vi "DOE Extract TCs.vi"(6 "Data Logger Type":T1=enum."Agilent", 8 "Error In":errorcluster, 9 "Agilent Array":dbl[](array[numeric]), 10 "TC Coefficients":T2, 11 "Kitchen Cluster in":T3) -> (0 "Error Out":errorcluster, 2 "TC Coefficients Out":T2, 3 "Kitchen Cluster out":T3, 4 "appended array":i32[](array[numeric]))   [LabVIEW 2018]
uses:
  Type Definitions/DOE Kitchen Control.ctl
  Utility/Type Definitions/UTILITY TC Coefficients.ctl
  Type Definitions/DOE Data Logger Type.ctl
  Utility/Type Definitions/UTILITY TC Coefficients Selector.ctl
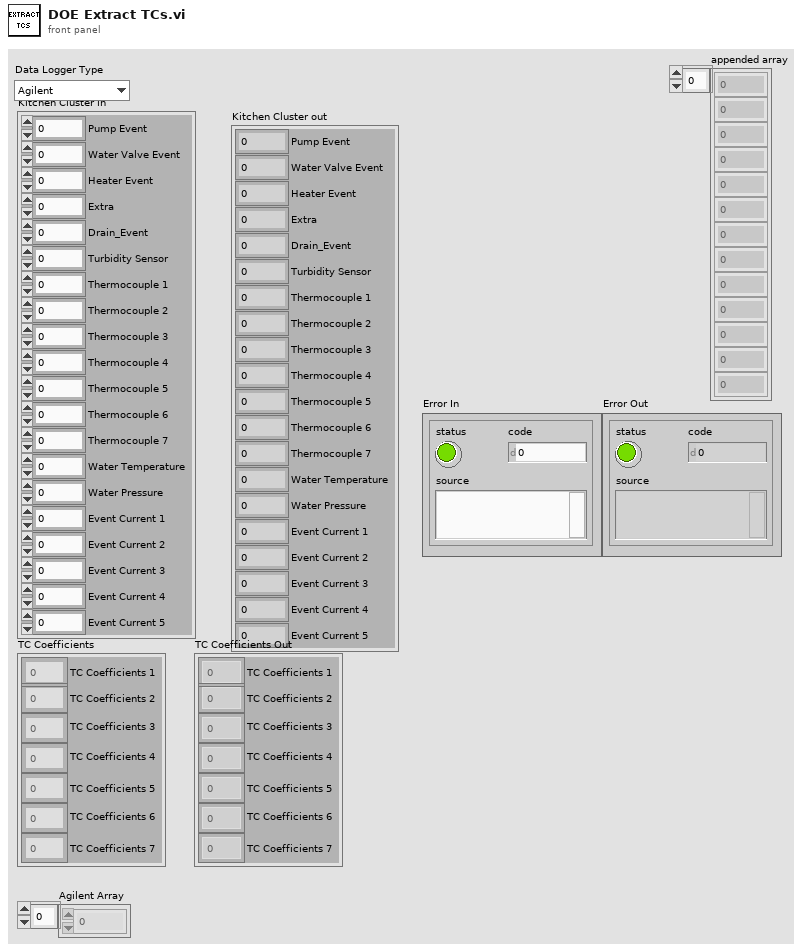
[diagram p1: front panel]
types:
  T1 = typedef "DOE Data Logger Type.ctl" = enum16{"MW100", "Agilent", "Agilent_Laurel_DC_Clamp"}
  T2 = typedef "UTILITY TC Coefficients.ctl" = cluster{"TC Coefficients 1":dbl[], "TC Coefficients 2":dbl[], "TC Coefficients 3":dbl[], "TC Coefficients 4":dbl[], "TC Coefficients 5":dbl[], "TC Coefficients 6":dbl[], "TC Coefficients 7":dbl[]}
  T3 = typedef "DOE Kitchen Control.ctl" = cluster{"Drain_Event":i16, "Pump Event":i16, "Water Valve Event":i16, "Heater Event":i16, "Extra":i16, "Turbidity Sensor":dbl, "Thermocouple 1":dbl, "Thermocouple 2":dbl, "Thermocouple 3":dbl, "Thermocouple 4":dbl, "Thermocouple 5":dbl, "Thermocouple 6":dbl, "Water Temperature":dbl, "Water Pressure":dbl, "Event Current 1":dbl, "Event Current 2":dbl, "Event Current 3":dbl, "Event Current 4":dbl, "Event Current 5":dbl, "Thermocouple 7":dbl}
  T4 = typedef "UTILITY TC Coefficients Selector.ctl" = enum16{"TC1", "TC2", "TC3", "TC4", "TC5", "TC6", "TC7"}
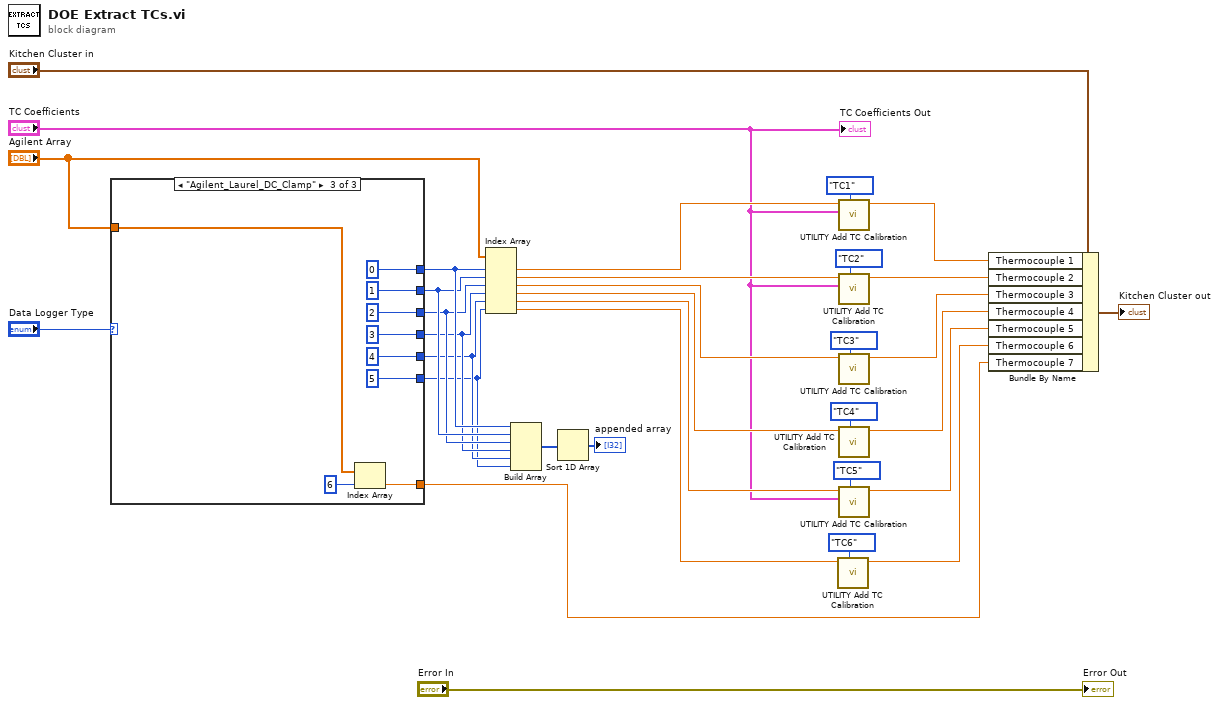
[diagram p0: block diagram]
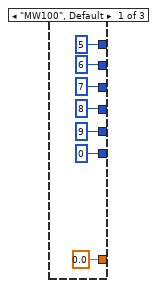
[diagram p2: hidden frame]
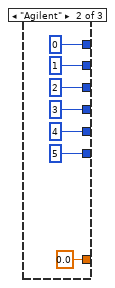
[diagram p3: hidden frame]
diagram:
  n1 = case shown="\"Agilent_Laurel_DC_Clamp\"" "Data Logger Type" {
    tunnel: [0 ("index") 5 ("index") 5 ("index")] -> w5
    tunnel: [9 ("index") 4 ("index") 4 ("index")] -> w6
    tunnel: [8 ("index") 3 ("index") 3 ("index")] -> w7
    tunnel: [7 ("index") 2 ("index") 2 ("index")] -> w8
    tunnel: [6 ("index") 1 ("index") 1 ("index")] -> w9
    tunnel: [5 ("index") 0 ("index") 0 ("index")] -> w10
    tunnel: "Agilent Array" -> [_ _ w49]
    tunnel: [0.0 ("Numeric") 0.0 ("Numeric") w48] -> w1
    frame "MW100", Default {
    }
    frame "Agilent" {
    }
    frame "Agilent_Laurel_DC_Clamp" {
      n2 = Index Array(array=w49, index=6) -> (element=w48:dbl)
    }
  }
  n3 = Index Array(array="Agilent Array", index #1=w10, index #2=w9, index #3=w8, index #4=w7, index #5=w6, index #6=w5) -> (element #1=w20:dbl, element #2=w21:dbl, element #3=w22:dbl, element #4=w23:dbl, element #5=w24:dbl, element #6=w25:dbl)
  n4 = Build Array(w10, w9, w8, w7, w6, w5) -> (w4:i32[])
  n5 = Sort 1D Array(array=w4) -> (sorted array=→"appended array":i32[])
  n6 = call "UTILITY Add TC Calibration.vi"("Enum"=UTILITY_TC_Coefficients_Selector."TC6", "Non Cal Temp"=w25) -> ("Calibrated Temp"=w32:dbl)  [unwired: 9 in]
  n7 = call "UTILITY Add TC Calibration.vi"("Enum"=UTILITY_TC_Coefficients_Selector."TC1", "TC Coefficients"="TC Coefficients", "Non Cal Temp"=w20) -> ("Calibrated Temp"=w27:dbl)  [unwired: 8 in]
  n8 = call "UTILITY Add TC Calibration.vi"("Enum"=UTILITY_TC_Coefficients_Selector."TC2", "TC Coefficients"="TC Coefficients", "Non Cal Temp"=w21) -> ("Calibrated Temp"=w28:dbl)  [unwired: 8 in]
  n9 = call "UTILITY Add TC Calibration.vi"("Enum"=UTILITY_TC_Coefficients_Selector."TC3", "Non Cal Temp"=w22) -> ("Calibrated Temp"=w29:dbl)  [unwired: 9 in]
  n10 = call "UTILITY Add TC Calibration.vi"("Enum"=UTILITY_TC_Coefficients_Selector."TC4", "Non Cal Temp"=w23) -> ("Calibrated Temp"=w30:dbl)  [unwired: 9 in]
  n11 = call "UTILITY Add TC Calibration.vi"("Enum"=UTILITY_TC_Coefficients_Selector."TC5", "TC Coefficients"="TC Coefficients", "Non Cal Temp"=w24) -> ("Calibrated Temp"=w31:dbl)  [unwired: 8 in]
  n12 = Bundle By Name(cluster="Kitchen Cluster in", "Thermocouple 1"=w27, "Thermocouple 2"=w28, "Thermocouple 3"=w29, "Thermocouple 4"=w30, "Thermocouple 5"=w31, "Thermocouple 6"=w32, "Thermocouple 7"=w1) -> (→"Kitchen Cluster out":T3)
  "Error Out" <- "Error In"
  "TC Coefficients Out" <- "TC Coefficients"
